vi "Create.vi"(8 "error in (no error)":errorcluster, 10 "Analog_Configuration_Parameters":T1) -> (0 "error out":errorcluster, 3 "Analog Output out":refnum<class "Analog Output.lvclass">)   [LabVIEW 2021, in "Analog Output.lvlib" / "Analog Output.lvclass"]
uses:
  Analog Output.lvclass
  Analog Output.lvclass/Analog Output.ctl
  <vilib>/DAQmx/write.llb/DAQmx Write (Analog DBL 1Chan 1Samp).vi
  <vilib>/DAQmx/create/channels.llb/DAQmx Create Channel (AO-Voltage-Basic).vi
  Utilities/Analog Configuration Parameters.ctl
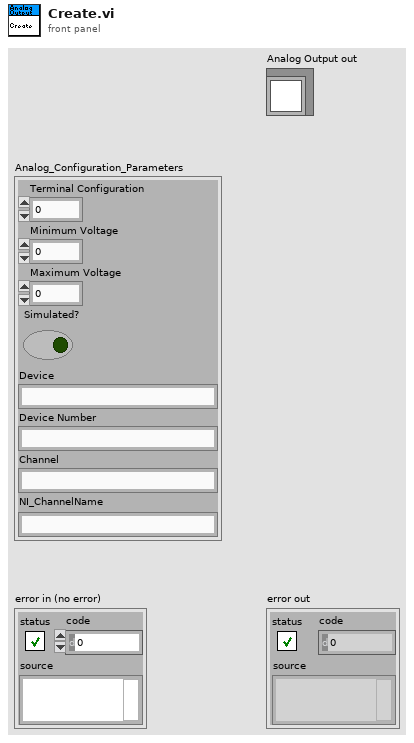
[diagram p1: front panel]
types:
  T1 = typedef "Analog Configuration Parameters.ctl" = cluster{"Terminal Configuration":i32, "Minimum Voltage":dbl, "Maximum Voltage":dbl, "Simulated?":bool, "Device":string, "Device Number":string, "Channel":string, "NI_ChannelName":string}
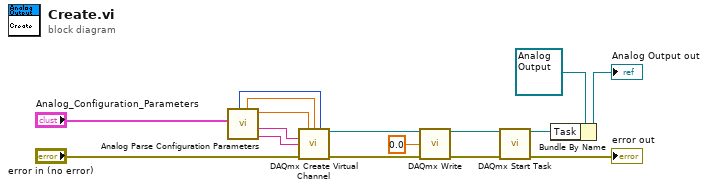
[diagram p0: block diagram]
diagram:
  n1 = call "Analog Parse Configuration Parameters.vi"("Analog Configuration Parameters"="Analog_Configuration_Parameters") -> ("name to assign"=w5:string, "physical channels"=w6:string, "Maximum Voltage"=w7:dbl, "Minimum Voltage"=w8:dbl, "Terminal Configuration"=w9:i32)  [unwired: 6 in]
  n2 = call-poly <vilib>:"DAQmx Create Virtual Channel.vi"("maximum value"=w7, "minimum value"=w8, "output terminal configuration"=w9, "physical channels"=w6, "name to assign"=w5, "error in"="error in (no error)") -> ("task out"=w16:refnum<k21>, "error out"=w15:errorcluster)  [unwired: 8 in]
  n3 = call-poly <vilib>:"DAQmx Write.vi"("task/channels in"=w16, "data"=0.0, "error in"=w15) -> ("task out"=w14:refnum<k21>, "error out"=w13:errorcluster)  [unwired: 10 in, 1 out]
  n4 = call <vilib>:"DAQmx Start Task.vi"("task/channels in"=w14, "error in"=w13) -> ("task out"=w12:refnum<k21>, "error out"=→"error out":errorcluster)  [unwired: 12 in]
  n5 = Bundle By Name(cluster=refnum<class "Analog Output.lvclass"> refnum ("Output out"), "Task"=w12) -> (→"Analog Output out":refnum<class "Analog Output.lvclass">)
